vi "Index Array (Numeric).vi"(8 "error in (no error)":errorcluster, 9 "index":i32, 10 "JSON Array in":refnum<class "JSON Array.lvclass">) -> (0 "error out":errorcluster, 1 "JSON Numeric":refnum<class "JSON Numeric.lvclass">)   [LabVIEW 2015, in "LVJSON.lvlib" / "JSON Array.lvclass"]
uses:
  JSON Array.lvclass
  JSON Numeric/JSON Numeric.lvclass
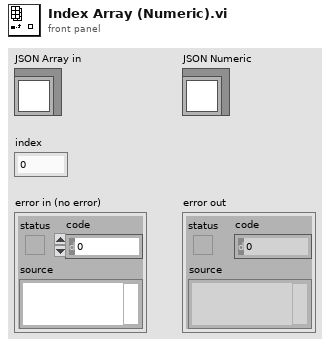
[diagram p1: front panel]
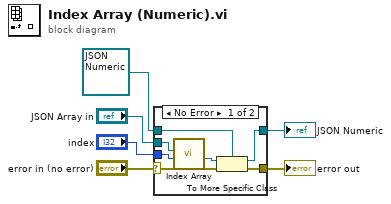
[diagram p0: block diagram]
diagram:
  n1 = case shown="No Error" "error in (no error)" {
    selector: "error in (no error)" -> [w7 w15]
    tunnel: [w12 w15] -> w5
    tunnel: "JSON Array in" -> [w8 _]
    tunnel: "index" -> [w11 _]
    tunnel: [w13 w14] -> w1
    tunnel: refnum<class "JSON Numeric.lvclass"> refnum ("target class") -> [w10 w14]
    frame No Error {
      n2 = call "Index Array.vi"("index"=w11, "JSON Array in"=w8) -> ("JSON Data"=w9:refnum<class "JSON Datatype.lvclass">)  [unwired: 9 in]
      n3 = To More Specific Class(target class=w10, reference=w9, error in=w7) -> (specific class reference=w13:refnum<class "JSON Numeric.lvclass">, error out=w12:errorcluster)
    }
    frame Error {
    }
  }
  "error out" <- w5
  "JSON Numeric" <- w1
